vi "播放器.vi"() -> ()   [LabVIEW 2014]
panel:
  in  "WindowsMediaPlayer":refnum<k7>(container)
  in  "停止":bool
  in  "路径":path
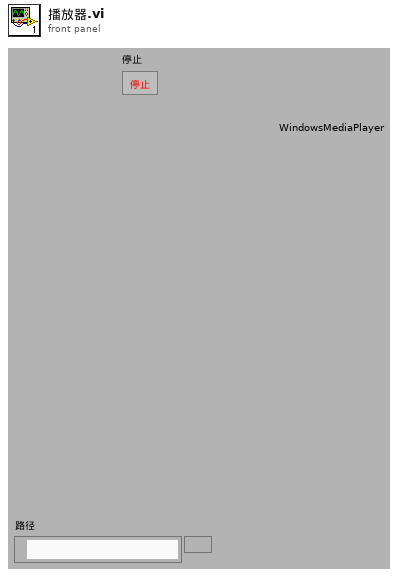
[diagram p1: front panel]
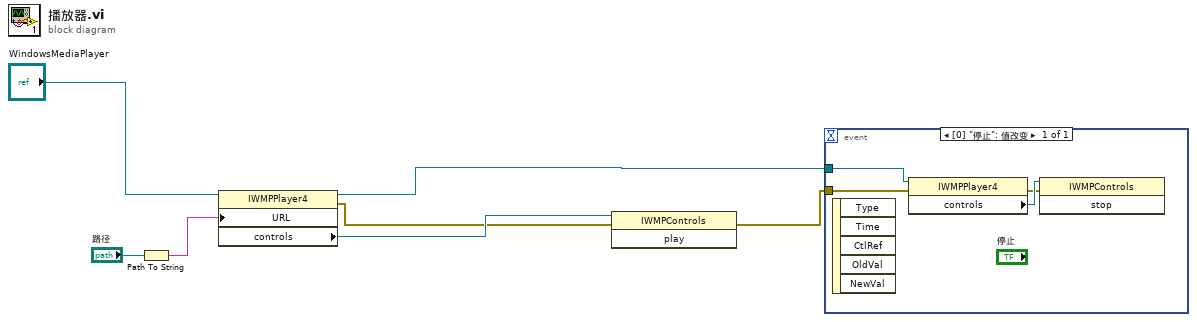
[diagram p0: block diagram]
diagram:
  n1 = Path To String(path="路径") -> (string=w6:string)
  n2 = property class="IWMPPlayer4"(reference="WindowsMediaPlayer", "URL"=w6) -> (reference out=w3:refnum<k7>, error out=w4:errorcluster, "controls"=w5:refnum<k7>)  [unwired: 1 in]
  n3 = invoke class="IWMPControls" method="play"(reference=w5, error in=w4) -> (error out=w2:errorcluster)  [unwired: 1 in, 2 out]
  n4 = event shown="[0] \"停止\": 值改变" {
    selector: _ -> [_]
    dyn-events: _ -> [_]
    timeout: _ -> [_]
    tunnel: w3 -> [w11]
    tunnel: w2 -> [w10]
    event "停止": Value Change {
      n5 = event-data() -> ()  [unwired: 1 in, 5 out]
      n6 = property class="IWMPPlayer4"(reference=w11, error in=w10) -> (error out=w8:errorcluster, "controls"=w9:refnum<k7>)  [unwired: 1 out]
      n7 = invoke class="IWMPControls" method="stop"(reference=w9, error in=w8) -> ()  [unwired: 1 in, 3 out]
    }
  }
